vi "Illumination Tests.vi"(0 "Test Number":i32, 5 "FileName":string="TestImage", 7 "Pixel Offset":i32, 9 "Pixel Average":i32) -> (1 "Hor Max":sgl format="%.2g", 2 "Vert Max":sgl format="%#.2g", 3 "Gray Level Intensity":T2 {"Standard  Deviation" format="%.2f"; "Mean Intensity" format="%.2f"; "Maximum Intensity" format="%.2f"; "Minimum Intensity" format="%.2f"}, 4 "Mean Intensity":sgl, 6 "Horz Ratio":sgl format="%#.2g", 10 "Vert Ratio":sgl format="%#.2g", 12 "Horz Min":sgl format="%.2g", 14 "Vert Min":sgl format="%#.2g", 15 "error out":errorcluster)   [LabVIEW 2014]
uses:
  <vilib>/vision/NI_Vision_Development_Module.lvlib
panel:
  out "Image":T1(plugin-control)
  out "Vertical Averages":sgl[](array[numeric]) format="%#.2g"
  out "Horizontal Averages":sgl[](array[numeric]) format="%#.2g"
  in  "error in (no error)":errorcluster
  # "0 = Center Illumination Brightness\n1 = Uniformity"
  # "UNIFORMITY"
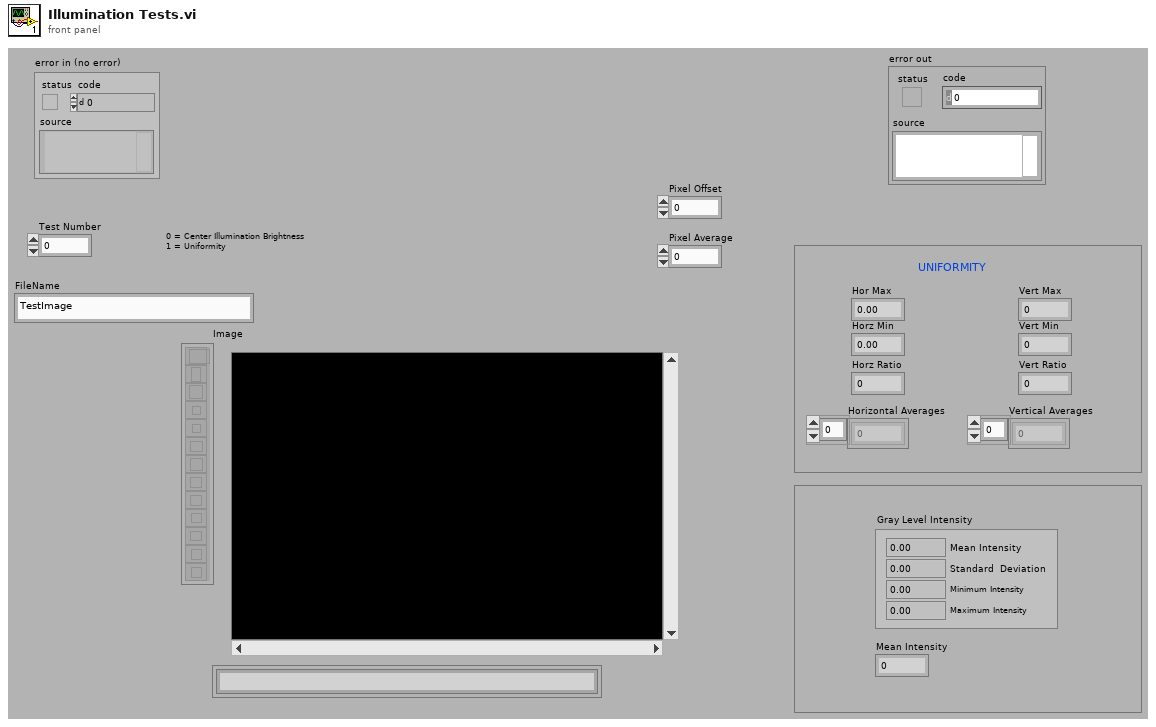
[diagram p1: front panel]
types:
  T1 = typedef "IMAQ Image.ctl" = refnum<image>
  T2 = cluster{"Mean Intensity":sgl, "Standard  Deviation":sgl, "Minimum Intensity":sgl, "Maximum Intensity":sgl}
  T3 = typedef "IMAQ Rectangle" = cluster{"Left":i32, "Top":i32, "Right":i32, "Bottom":i32, "Rotation":dbl}
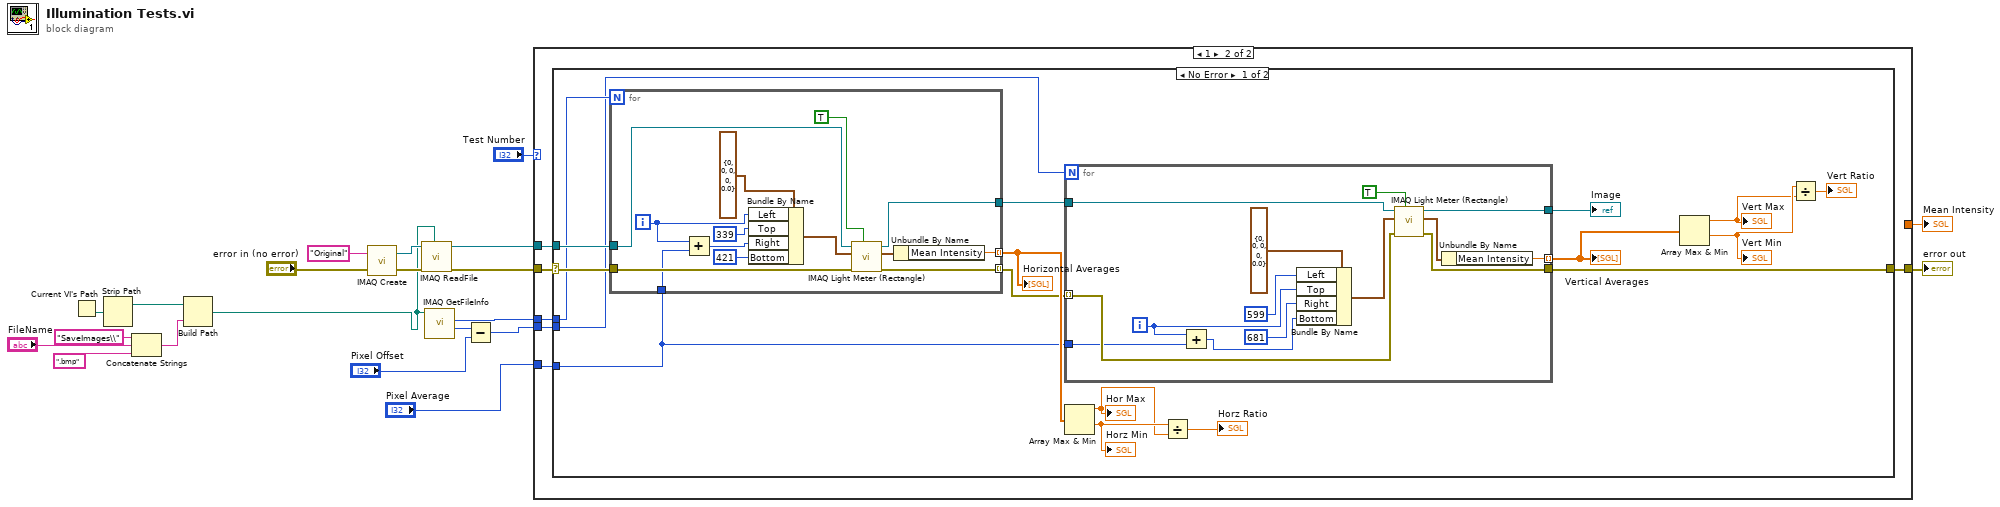
[diagram p0: block diagram]
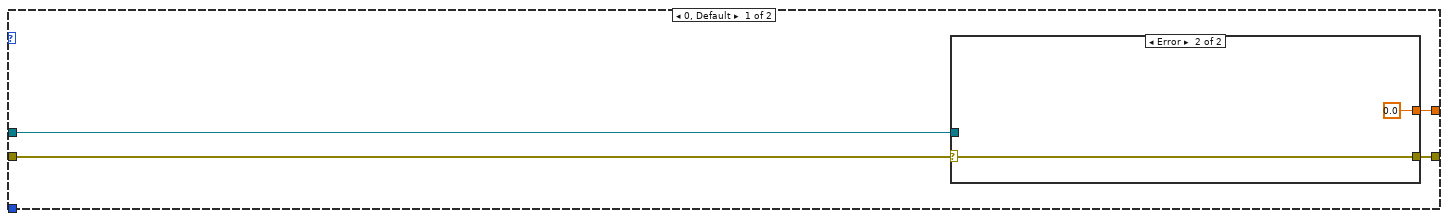
[diagram p2: hidden frame]
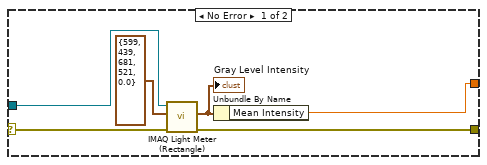
[diagram p3: hidden frame]
diagram:
  n1 = Current VI's Path() -> (path=w8:path)
  n2 = Strip Path(path=w8) -> (stripped path=w7:path)  [unwired: 1 out]
  n3 = Concatenate Strings("SaveImages\\" ("string"), "FileName", ".bmp" ("string")) -> (w6:string)
  n4 = Build Path(base path=w7, name or relative path=w6) -> (appended path=w2:path)
  n5 = call "IMAQ Create"("Image Name"="Original", "error in (no error)"="error in (no error)") -> ("New Image"=w20:T1, "error out"=w17:errorcluster)  [unwired: 3 in]
  n6 = call "IMAQ ReadFile"("File Path"=w2, "error in (no error)"=w17, "Image"=w20) -> ("error out"=w16:errorcluster, "Image Out"=w19:T1)  [unwired: 4 in, 3 out]
  n7 = call "IMAQ GetFileInfo"("File Path"=w2) -> ("Y Resolution"=w10:i32, "X Resolution"=w12:i32)  [unwired: 4 in, 5 out]
  n8 = Subtract(x=w10, y="Pixel Offset") -> (x-y=w11:i32)
  n9 = case shown="1" "Test Number" {
    tunnel: w19 -> [w25 w37]
    tunnel: w16 -> [w24 w39]
    tunnel: [w23 _] -> w15
    tunnel: [w22 w38] -> w14
    tunnel: w12 -> [_ w36]
    tunnel: w11 -> [_ w35]
    tunnel: "Pixel Average" -> [_ w34]
    frame 0, Default {
      n10 = case shown="Error" w24 {
        selector: w24 -> [w26 w32]
        tunnel: w25 -> [w30 _]
        tunnel: [w28 sgl 0.0 ("Mean Intensity")] -> w23
        tunnel: [w27 w32] -> w22
        frame No Error {
          n11 = call "IMAQ Light Meter (Rectangle)"("error in (no error)"=w26, "Rectangle"=T3 {"Left"=599, "Top"=439, "Right"=681, "Bottom"=521, "Rotation"=0.0}, "Image"=w30) -> ("error out"=w27:errorcluster, "Gray Level Intensities"=w29:T2)  [unwired: 4 in, 3 out]
          "Gray Level Intensity" <- w29
          n12 = Unbundle By Name(w29) -> ("Mean Intensity"=w28:sgl)
        }
        frame Error {
        }
      }
    }
    frame 1 {
      n13 = case shown="No Error" w39 {
        selector: w39 -> [w47 w85]
        tunnel: [w46 w85] -> w38
        tunnel: w37 -> [w43 _]
        tunnel: w36 -> [w42 _]
        tunnel: w35 -> [w41 _]
        tunnel: w34 -> [w40 _]
        frame No Error {
          n14 = for {
            N: w42 -> [_]
            tunnel: [w77] -> w56 mode=indexing
            tunnel: w43 -> [w75]
            tunnel: [w74] -> w48 mode=indexing
            tunnel: w47 -> [w73]
            tunnel: [w72] -> w45
            tunnel: w40 -> [w71]
            i -> [w82]
            n15 = Add(x=w82, y=w71) -> (x+y=w81:i32)
            n16 = Bundle By Name(cluster=T3 {"Left"=0, "Top"=0, "Right"=0, "Bottom"=0, "Rotation"=0.0} ("Rectangle"), "Left"=w82, "Top"=339, "Right"=w81, "Bottom"=421) -> (w79:T3)
            n17 = call "IMAQ Light Meter (Rectangle)"("Show Search Area"=TRUE, "error in (no error)"=w73, "Rectangle"=w79, "Image"=w75) -> ("error out"=w74:errorcluster, "Gray Level Intensities"=w78:T2, "Image Out"=w72:T1)  [unwired: 3 in, 2 out]
            n18 = Unbundle By Name(w78) -> ("Mean Intensity"=w77:sgl)
          }
          "Horizontal Averages" <- w56
          n19 = for {
            N: w41 -> [_]
            tunnel: [w67] -> w55 mode=indexing
            tunnel: [w66] -> w46
            tunnel: w48 -> [w60] mode=indexing
            tunnel: w45 -> [w59]
            tunnel: [w58] -> w44
            tunnel: w40 -> [w57]
            i -> [w63]
            n20 = Add(x=w63, y=w57) -> (x+y=w61:i32)
            n21 = Bundle By Name(cluster=T3 {"Left"=0, "Top"=0, "Right"=0, "Bottom"=0, "Rotation"=0.0} ("Rectangle"), "Left"=599 ("Top"), "Top"=w63, "Right"=681 ("Bottom"), "Bottom"=w61) -> (w69:T3)
            n22 = call "IMAQ Light Meter (Rectangle)"("Show Search Area"=TRUE, "error in (no error)"=w60, "Rectangle"=w69, "Image"=w59) -> ("error out"=w66:errorcluster, "Gray Level Intensities"=w68:T2, "Image Out"=w58:T1)  [unwired: 3 in, 2 out]
            n23 = Unbundle By Name(w68) -> ("Mean Intensity"=w67:sgl)
          }
          "Vertical Averages" <- w55
          "Image" <- w44
          n24 = Array Max & Min(array=w56) -> (max value=w51:sgl, min value=w52:sgl)  [unwired: 2 out]
          "Hor Max" <- w51
          "Horz Min" <- w52
          n25 = Divide(x=w52, y=w51) -> (x/y=→"Horz Ratio":sgl)
          n26 = Array Max & Min(array=w55) -> (max value=w53:sgl, min value=w54:sgl)  [unwired: 2 out]
          "Vert Max" <- w53
          "Vert Min" <- w54
          n27 = Divide(x=w54, y=w53) -> (x/y=→"Vert Ratio":sgl)
        }
        frame Error {
        }
      }
    }
  }
  "Mean Intensity" <- w15
  "error out" <- w14
